vi "Simulated Device Page.vi"(8 "error in (no error)":errorcluster, 11 "Node Ptr":T1 format="%.0x") -> (0 "error out":errorcluster)   [LabVIEW 2023, in "J1939 Addon System Explorer.lvlib"]
uses:
  J1939 Addon System Explorer.lvlib
  <vilib>/NI VeriStand/Custom Device API/Custom Device Item Ref.ctl
  Addon Shared/SubVIs/Constants.vi
  <vilib>/NI VeriStand/Custom Device API/Custom Device API.lvlib
  Addon Shared/J1939 Addon Shared.lvlib
panel:
  in  "Force SA":bool
  in  "Include DA":bool
  in  "Settings":cluster{"Section Name":string}={"Section Name"="Address Settings"}
  in  "J1939 Name":u64 format="%.0x"
  in  "J1939 Network Address":u8 format="%.0x"
  in  "Description":string
  in  "Name":string
  in  "SHDocVw.IWebBrowser2":refnum<k7>(container)
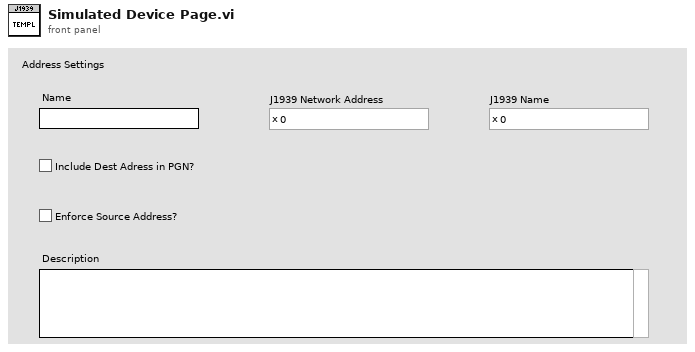
[diagram p1: front panel]
types:
  T1 = typedef "Custom Device API.lvlib/Custom Device Item Ref.ctl" = u64
  T2 = typedef "J1939 Addon Shared.lvlib/Monitor Settings.ctl" = cluster{"Address":u8, "Name":u64, "Include DA":bool, "Force SA":bool}
  T3 = typedef "Custom Device API.lvlib/Custom Device Item Info.ctl" = cluster{"Name":string, "Is Channel":bool, "GUID":string, "Is Waveform":bool}
  T4 = typedef "Custom Device API.lvlib/Custom Device Commands.ctl" = enum16{"Default", "Item renamed", "Shutdown", "Dynamic button pressed"}
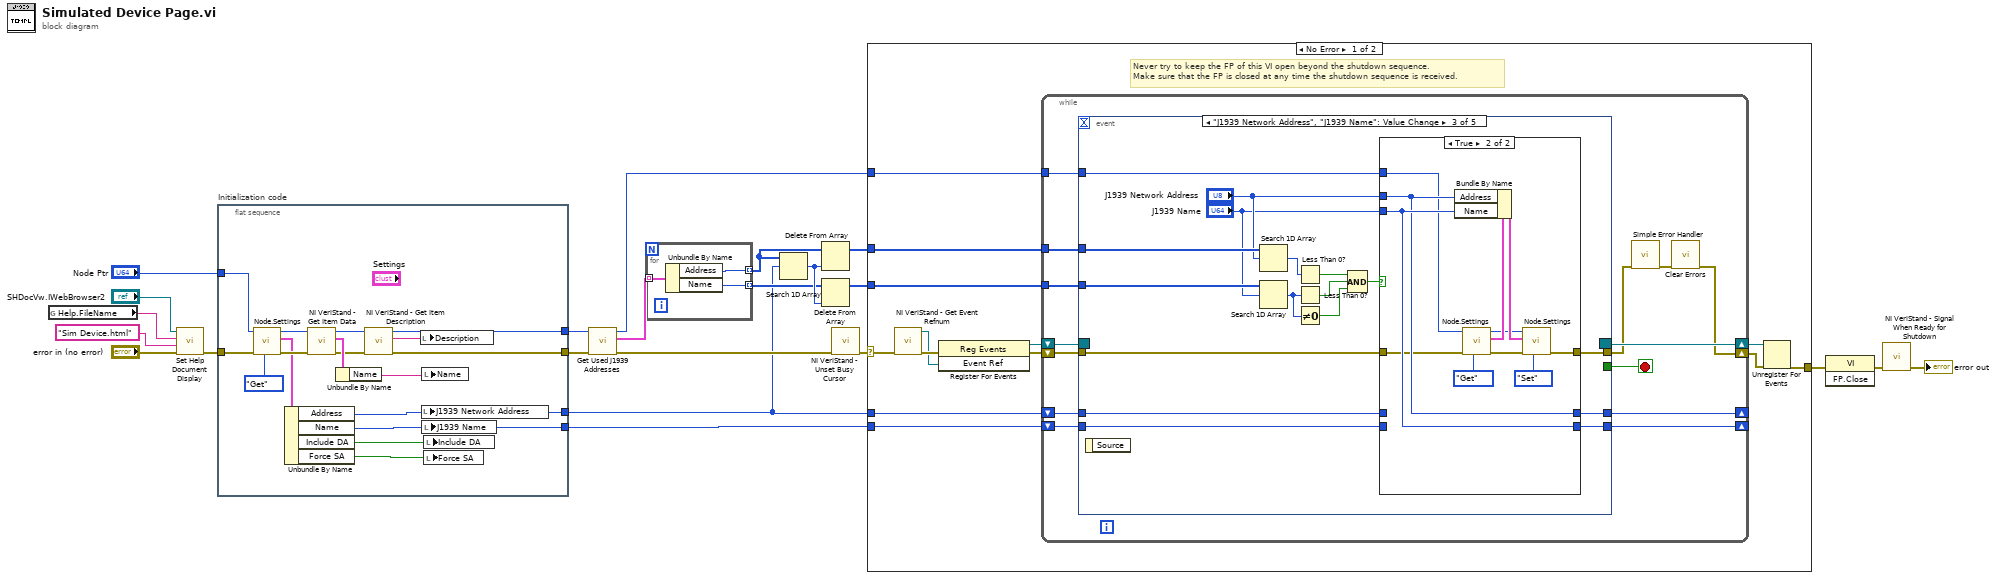
[diagram p0: block diagram]
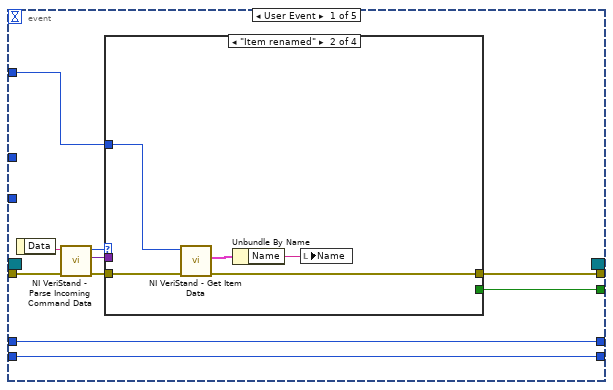
[diagram p2: hidden frame]
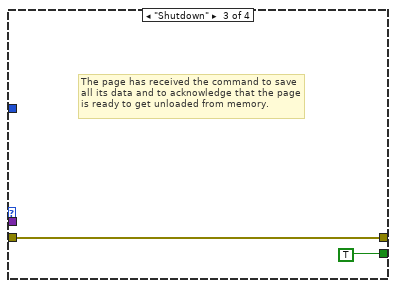
[diagram p4: hidden frame]
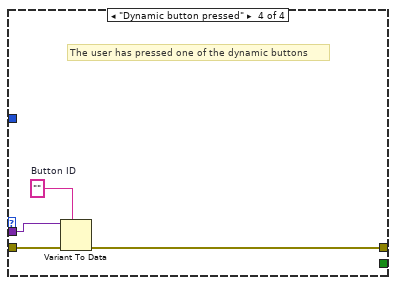
[diagram p5: hidden frame]
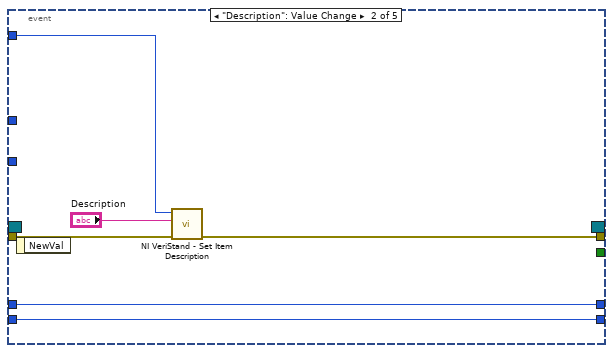
[diagram p6: hidden frame]
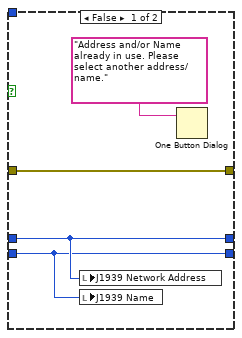
[diagram p7: hidden frame]
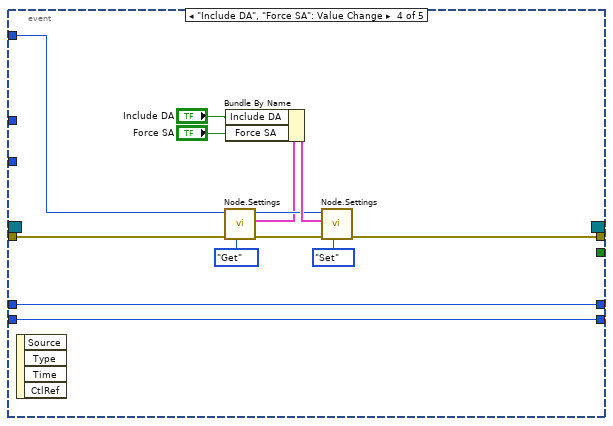
[diagram p8: hidden frame]
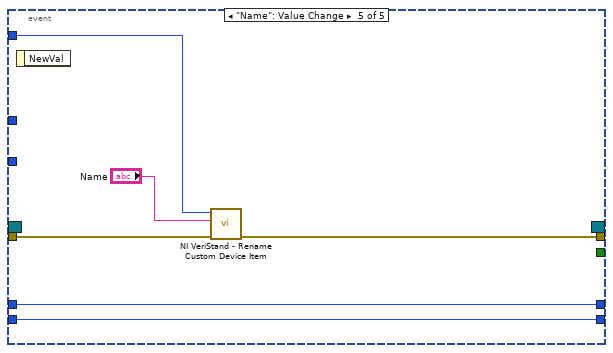
[diagram p9: hidden frame]
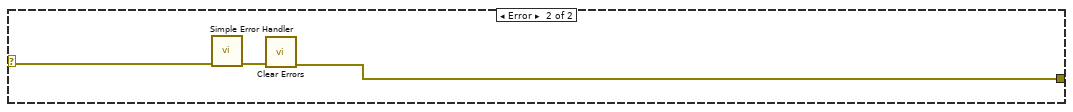
[diagram p10: hidden frame]
diagram:
  n1 = global read "Constants.vi" "Help.FileName"() -> (w1:string)
  n2 = call "Set Help Document Display.vi"("error in (no error)"="error in (no error)", "HTML File"="Sim Device.html", "Main CHM File"=w1, "SHDocVw.IWebBrowser2"="SHDocVw.IWebBrowser2") -> ("error out"=w14:errorcluster)  [unwired: 7 in]
  n3 = flat-sequence "Initialization code" {
    tunnel: w14 -> [w32]
    tunnel: "Node Ptr" -> [w31]
    tunnel: [w36] -> w12
    tunnel: [w34] -> w10
    tunnel: [w27] -> w4
    tunnel: [w26] -> w9
    frame #0 {
      n4 = call "Node.Settings.vi"("Action"=enum8{"Get", "Set"}."Get", "error in (no error)"=w32, "Item Ref in"=w31) -> ("error out"=w29:errorcluster, "Node.Settings"=w28:T2, "Item Ref out"=w30:T1)  [unwired: 6 in]
      n5 = Unbundle By Name(w28) -> ("Address"=w27:u8, "Name"=w26:u64, "Include DA"=w24:bool, "Force SA"=w23:bool)
      n6 = call <vilib>:"NI VeriStand - Get Item Data.vi"("error in (no error)"=w29, "Item Ref in"=w30) -> ("error out"=w37:errorcluster, "Item Info"=w39:T3, "Item Ref out"=w35:T1)  [unwired: 7 out]
      n7 = Unbundle By Name(w39) -> ("Name"=w38:string)
      n8 = call <vilib>:"NI VeriStand - Get Item Description.vi"("error in (no error)"=w37, "Item Ref in"=w35) -> ("error out"=w36:errorcluster, "Description"=w33:string, "Item Ref out"=w34:T1)  [unwired: 6 in, 1 out]
      n9 = local write "Description"(w33) -> ()
      n10 = local write "J1939 Network Address"(w27) -> ()
      n11 = local write "Name"(w38) -> ()
      n12 = local write "J1939 Name"(w26) -> ()
      n13 = local write "Include DA"(w24) -> ()
      n14 = local write "Force SA"(w23) -> ()
    }
  }
  n15 = call "Get Used J1939 Addresses.vi"("error in (no error)"=w12, "Node Ptr"=w10) -> ("error out"=w13:errorcluster, "Nodes"=w5:T2[], "Item Ref out"=w11:T1)  [unwired: 7 in]
  n16 = for {
    tunnel: w5 -> [w42] mode=indexing
    tunnel: [w41] -> w8 mode=indexing
    tunnel: [w40] -> w6 mode=indexing
    n17 = Unbundle By Name(w42) -> ("Address"=w41:u8, "Name"=w40:u64)
  }
  n18 = Search 1D Array(1D array=w8, element=w4) -> (index of element=w7:i32)  [unwired: 1 in]
  n19 = Delete From Array(array=w8, index=w7) -> (array with subset deleted=w3:u8[])  [unwired: 1 in, 1 out]
  n20 = Delete From Array(array=w6, index=w7) -> (array with subset deleted=w2:u64[])  [unwired: 1 in, 1 out]
  n21 = call <vilib>:"NI VeriStand - Unset Busy Cursor.vi"("error in (no error)"=w13) -> ("error out"=w18:errorcluster)  [unwired: 10 out]
  n22 = case shown="No Error" w18 {
    selector: w18 -> [w47 w151]
    tunnel: [w52 w149] -> w22
    tunnel: w11 -> [w48 _]
    tunnel: w4 -> [w46 _]
    tunnel: w9 -> [w45 _]
    tunnel: w3 -> [w44 _]
    tunnel: w2 -> [w43 _]
    frame No Error {
      # "Never try to keep the FP of this VI open beyond the shutdown sequence.\nMake sure that the FP is closed at any time the shutdown sequence is received."
      n23 = call <vilib>:"NI VeriStand - Get Event Refnum.vi"("error in (no error)"=w47) -> ("error out"=w55:errorcluster, "Event Ref"=w51:refnum<user-event>)  [unwired: 9 out]
      n24 = register-events(error in=w55, w51) -> (reference out=w49:refnum<event-registration>, error out=w50:errorcluster)  [unwired: 1 in]
      n25 = while {
        tunnel: w48 -> [w65]
        shift-right: [w62] -> w53
        shift-left: w50 -> [w68]
        shift-right: [w69] -> w54
        shift-left: w49 -> [w67]
        tunnel: w44 -> [w59]
        tunnel: w43 -> [w58]
        shift-right: [w57] -> _
        shift-left: w46 -> [w61]
        shift-right: [w56] -> _
        shift-left: w45 -> [w60]
        stop <- w66 stop-if-true
        n26 = event shown="[2] \"J1939 Network Address\", \"J1939 Name\": Value Change" {
          selector: w67 -> [_ _ _ _ _]
          dyn-events: [_ _ _ _ _] -> w69
          timeout: _ -> [_ _ _ _ _]
          tunnel: w68 -> [w79 w97 w114 w135 w148]
          tunnel: [w75 _ _ _ _] -> w66
          tunnel: [w74 w94 w113 w142 w146] -> w64
          tunnel: w65 -> [w73 w95 w112 w134 w147]
          tunnel: w61 -> [w70 w92 w111 w138 w143]
          tunnel: w60 -> [w71 w93 w110 w139 w144]
          tunnel: w59 -> [_ _ w104 _ _]
          tunnel: w58 -> [_ _ w103 _ _]
          tunnel: [w70 w92 w99 w138 w143] -> w57
          tunnel: [w71 w93 w98 w139 w144] -> w56
          event User Event {
            n27 = event-data() -> ("Data"=w78:string)  [unwired: 1 out]
            n28 = call <vilib>:"NI VeriStand - Parse Incoming Command Data.vi"("error in (no error)"=w79, "Incoming data"=w78) -> ("error out"=w77:errorcluster, "Outgoing data"=w72:variant, "Action"=w76:T4)  [unwired: 7 out]
            n29 = case shown="\"Item renamed\"" w76 {
              tunnel: w77 -> [w80 w83 w86 w91]
              tunnel: [_ _ TRUE _] -> w75
              tunnel: [w80 w81 w86 w88] -> w74
              tunnel: w73 -> [_ w82 _ _]
              tunnel: w72 -> [_ _ _ w90]
              frame "Default", Default {
              }
              frame "Item renamed" {
                n30 = call <vilib>:"NI VeriStand - Get Item Data.vi"("error in (no error)"=w83, "Item Ref in"=w82) -> ("error out"=w81:errorcluster, "Item Info"=w84:T3)  [unwired: 8 out]
                n31 = Unbundle By Name(w84) -> ("Name"=w85:string)
                n32 = local write "Name"(w85) -> ()
              }
              frame "Shutdown" {
                # "The page has received the command to save all its data and to acknowledge that the page is ready to get unloaded from memory."
              }
              frame "Dynamic button pressed" {
                w89 = ""  # Button ID
                # "The user has pressed one of the dynamic buttons"
                n33 = Variant To Data(error in=w91, type=w89, Variant=w90) -> (error out=w88:errorcluster)  [unwired: 1 out]
              }
            }
          }
          event "Description": Value Change {
            n34 = event-data() -> ()  [unwired: 2 out]
            n35 = call <vilib>:"NI VeriStand - Set Item Description.vi"("error in (no error)"=w97, "Description"="Description", "Item Ref in"=w95) -> ("error out"=w94:errorcluster)  [unwired: 6 in, 2 out]
          }
          event "J1939 Network Address", "J1939 Name": Value Change {
            n36 = event-data() -> ()  [unwired: 2 out]
            n37 = Search 1D Array(1D array=w104, element="J1939 Network Address") -> (index of element=w107:i32)  [unwired: 1 in]
            n38 = Search 1D Array(1D array=w103, element="J1939 Name") -> (index of element=w106:i32)  [unwired: 1 in]
            n39 = Less Than 0?(x=w107) -> (x < 0?=w109:bool)
            n40 = Less Than 0?(x=w106) -> (x < 0?=w108:bool)
            n41 = Not Equal To 0?(x=w106) -> (x != 0?=w105:bool)
            n42 = Compound Arithmetic op=AND(w109, w108, w105) -> (w100:bool)
            n43 = case shown="True" w100 {
              tunnel: "J1939 Name" -> [_ w128]
              tunnel: w114 -> [w118 w123]
              tunnel: [w118 w129] -> w113
              tunnel: w112 -> [_ w120]
              tunnel: "J1939 Network Address" -> [_ w127]
              tunnel: w111 -> [w116 _]
              tunnel: w110 -> [w115 _]
              tunnel: [w116 w127] -> w99
              tunnel: [w115 w128] -> w98
              frame False {
                n44 = local write "J1939 Network Address"(w116) -> ()
                n45 = local write "J1939 Name"(w115) -> ()
                n46 = One Button Dialog(message="Address and/or Name already in use. Please select another address/name.") -> ()  [unwired: 1 in, 1 out]
              }
              frame True {
                n47 = call "Node.Settings.vi"("Action"=enum8{"Get", "Set"}."Get", "error in (no error)"=w123, "Item Ref in"=w120) -> ("error out"=w122:errorcluster, "Node.Settings"=w121:T2, "Item Ref out"=w119:T1)  [unwired: 6 in]
                n48 = Bundle By Name(cluster=w121, "Address"=w127, "Name"=w128) -> (w126:T2)
                n49 = call "Node.Settings.vi"("Action"=enum8{"Get", "Set"}."Set", "error in (no error)"=w122, "Node.Settings"=w126, "Item Ref in"=w119) -> ("error out"=w129:errorcluster)  [unwired: 5 in, 2 out]
              }
            }
          }
          event "Include DA", "Force SA": Value Change {
            n50 = event-data() -> ()  [unwired: 5 out]
            n51 = call "Node.Settings.vi"("Action"=enum8{"Get", "Set"}."Get", "error in (no error)"=w135, "Item Ref in"=w134) -> ("error out"=w136:errorcluster, "Node.Settings"=w132:T2, "Item Ref out"=w133:T1)  [unwired: 6 in]
            n52 = Bundle By Name(cluster=w132, "Include DA"="Include DA", "Force SA"="Force SA") -> (w141:T2)
            n53 = call "Node.Settings.vi"("Action"=enum8{"Get", "Set"}."Set", "error in (no error)"=w136, "Node.Settings"=w141, "Item Ref in"=w133) -> ("error out"=w142:errorcluster)  [unwired: 5 in, 2 out]
          }
          event "Name": Value Change {
            n54 = event-data() -> ()  [unwired: 2 out]
            n55 = call <vilib>:"NI VeriStand - Rename Custom Device Item.vi"("error in (no error)"=w148, "New Name"="Name", "Item Ref in"=w147) -> ("error out"=w146:errorcluster)  [unwired: 1 in, 7 out]
          }
        }
        n56 = call <vilib>:"Simple Error Handler.vi"("error in (no error)"=w64) -> ("error out"=w63:errorcluster)  [unwired: 1 in, 7 out]
        n57 = call <vilib>:"Clear Errors.vi"("error in (no error)"=w63) -> ("error out"=w62:errorcluster)  [unwired: 1 in, 5 out]
      }
      n58 = Unregister For Events(event registration refnum=w54, error in=w53) -> (error out=w52:errorcluster)
    }
    frame Error {
      n59 = call <vilib>:"Simple Error Handler.vi"("error in (no error)"=w151) -> ("error out"=w150:errorcluster)  [unwired: 1 in, 7 out]
      n60 = call <vilib>:"Clear Errors.vi"("error in (no error)"=w150) -> ("error out"=w149:errorcluster)  [unwired: 1 in, 5 out]
    }
  }
  n61 = invoke class="VI" method="FP.Close"(error in=w22) -> (error out=w21:errorcluster)  [unwired: 2 in, 2 out]
  n62 = call <vilib>:"NI VeriStand - Signal When Ready for Shutdown.vi"("error in (no error)"=w21) -> ("error out"=→"error out":errorcluster)  [unwired: 10 out]
